vi "Lvi Create Task.vi"(7 "SEorDiff":u32, 8 "error in (no error)":errorcluster, 9 "SubSysIndex":u32, 10 "ChanType":u32, 11 "BoardName":string) -> (0 "error out":errorcluster, 2 "function return":u32(ring), 3 "TaskRef":i32)   [LabVIEW 2022 SP3, in "DtLvLink.lvlib"]
doc: "Calls directly into the entry points of the DLL of the Data Acq SDK to create one or more virtual channels, add them to a task, and configure the task with the specified settings. This VI is used by the higher-level VI, DtOLCreateTask."
uses:
  DtLvLink.lvlib
  <userlib>/LV-Link3/DtLvLink_64.dll
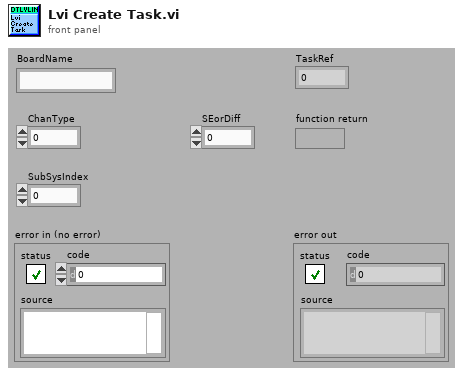
[diagram p1: front panel]
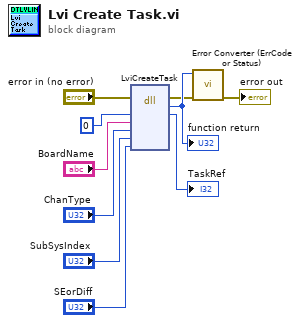
[diagram p0: block diagram]
diagram:
  n1 = dll-call lib="C:/Program Files/National Instruments/LabVIEW 2022/user.lib/LV-Link3/DtLvLink_64.*" fn="LviCreateTask"(error in="error in (no error)", "TaskRef"=0, "BoardName"="BoardName", "ChanType"="ChanType", "SubSysIndex"="SubSysIndex", "SEorDiff"="SEorDiff") -> (error out=w2:errorcluster, w10:u32, "TaskRef"=→"TaskRef":i32)  [unwired: 6 in, 1 out]
  "function return" <- w10
  n2 = call "Error Converter (ErrCode or Status).vi"("error in (no error)"=w2, "error code"=w10) -> ("error out"=→"error out":errorcluster)  [unwired: 9 in]
